vi "test_libssh2_sftp_readlink.vi"() -> ()   [LabVIEW 2017, in "integration_tests.lvlib"]
uses:
  integration_tests.lvlib
  libssh2/libssh2_sftp_symlink_ex.vi
  support/support.lvlib
  libssh2/libssh2.lvlib
  <vilib>/PNR/Transparent Assertions/Transparent Assertions/Transparent Assertions.lvlib
panel:
  out "error out":errorcluster
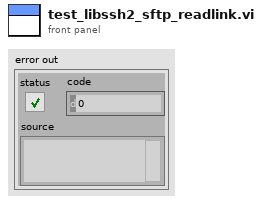
[diagram p1: front panel]
types:
  T1 = typedef "libssh2.lvlib/Session Refnum.ctl" = refnum<k1>
  T2 = typedef "libssh2.lvlib/SFTP Refnum.ctl" = refnum<k1>
  T3 = typedef "libssh2.lvlib/SFTP Handle Refnum.ctl" = refnum<k1>
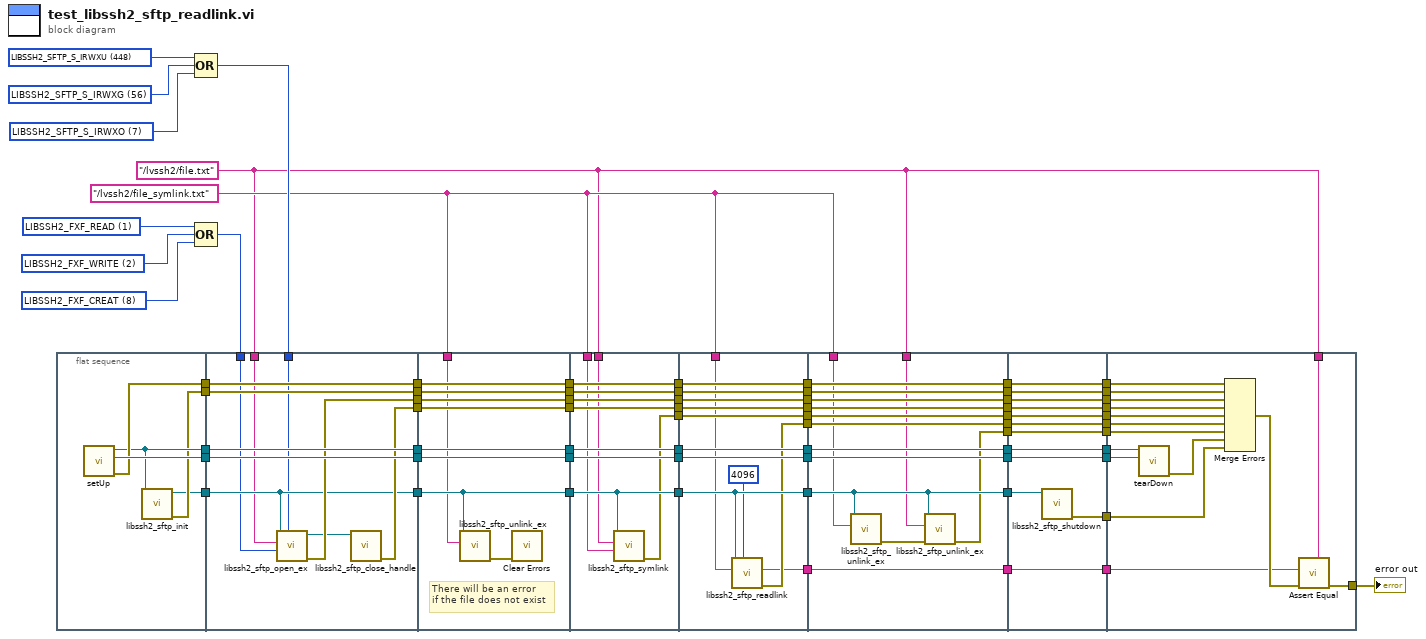
[diagram p0: block diagram]
diagram:
  w4 = "/lvssh2/file_symlink.txt" ("filename")
  w59 = u32 2 items=["LIBSSH2_FXF_READ"=1, "LIBSSH2_FXF_WRITE"=2, "LIBSSH2_FXF_APPEND"=4, "LIBSSH2_FXF_CREAT"=8, "LIBSSH2_FXF_TRUNC"=16, "LIBSSH2_FXF_EXCL"=32] ("flags")
  w60 = u32 1 items=["LIBSSH2_FXF_READ"=1, "LIBSSH2_FXF_WRITE"=2, "LIBSSH2_FXF_APPEND"=4, "LIBSSH2_FXF_CREAT"=8, "LIBSSH2_FXF_TRUNC"=16, "LIBSSH2_FXF_EXCL"=32] ("flags")
  w58 = u32 8 items=["LIBSSH2_FXF_READ"=1, "LIBSSH2_FXF_WRITE"=2, "LIBSSH2_FXF_APPEND"=4, "LIBSSH2_FXF_CREAT"=8, "LIBSSH2_FXF_TRUNC"=16, "LIBSSH2_FXF_EXCL"=32] ("flags")
  w3 = "/lvssh2/file.txt" ("filename")
  w62 = 7 items=["LIBSSH2_SFTP_S_IRWXU"=448, "LIBSSH2_SFTP_S_IRUSR"=256, "LIBSSH2_SFTP_S_IWUSR"=128, "LIBSSH2_SFTP_S_IXUSR"=64, "LIBSSH2_SFTP_S_IRWXG"=56, "LIBSSH2_SFTP_S_IRGRP"=32, "LIBSSH2_SFTP_S_IWGRP"=16, "LIBSSH2_SFTP_S_IXGRP"=8, "LIBSSH2_SFTP_S_IRWXO"=7, "LIBSSH2_SFTP_S_IROTH"=4, "LIBSSH2_SFTP_S_IWOTH"=2, "LIBSSH2_SFTP_S_IXOTH"=1] ("mode")
  w63 = 56 items=["LIBSSH2_SFTP_S_IRWXU"=448, "LIBSSH2_SFTP_S_IRUSR"=256, "LIBSSH2_SFTP_S_IWUSR"=128, "LIBSSH2_SFTP_S_IXUSR"=64, "LIBSSH2_SFTP_S_IRWXG"=56, "LIBSSH2_SFTP_S_IRGRP"=32, "LIBSSH2_SFTP_S_IWGRP"=16, "LIBSSH2_SFTP_S_IXGRP"=8, "LIBSSH2_SFTP_S_IRWXO"=7, "LIBSSH2_SFTP_S_IROTH"=4, "LIBSSH2_SFTP_S_IWOTH"=2, "LIBSSH2_SFTP_S_IXOTH"=1] ("mode")
  w64 = 448 items=["LIBSSH2_SFTP_S_IRWXU"=448, "LIBSSH2_SFTP_S_IRUSR"=256, "LIBSSH2_SFTP_S_IWUSR"=128, "LIBSSH2_SFTP_S_IXUSR"=64, "LIBSSH2_SFTP_S_IRWXG"=56, "LIBSSH2_SFTP_S_IRGRP"=32, "LIBSSH2_SFTP_S_IWGRP"=16, "LIBSSH2_SFTP_S_IXGRP"=8, "LIBSSH2_SFTP_S_IRWXO"=7, "LIBSSH2_SFTP_S_IROTH"=4, "LIBSSH2_SFTP_S_IWOTH"=2, "LIBSSH2_SFTP_S_IXOTH"=1] ("mode")
  n1 = flat-sequence {
    tunnel: [w73] -> w70
    tunnel: [w75] -> w69
    tunnel: [w74] -> w68
    tunnel: [w72] -> w66
    tunnel: [w71] -> w65
    tunnel: [w86] -> w38
    tunnel: [w85] -> w36
    tunnel: [w80] -> w34
    tunnel: [w84] -> w32
    tunnel: [w83] -> w30
    tunnel: [w82] -> w28
    tunnel: [w81] -> w26
    tunnel: w57 -> [w77]
    tunnel: w3 -> [w78]
    tunnel: w61 -> [w79]
    tunnel: w65 -> [w80]
    tunnel: w66 -> [w83]
    tunnel: w68 -> [w84]
    tunnel: w69 -> [w85]
    tunnel: w70 -> [w86]
    tunnel: w38 -> [w95]
    tunnel: [w95] -> w37
    tunnel: w36 -> [w94]
    tunnel: [w94] -> w35
    tunnel: w34 -> [w88]
    tunnel: [w88] -> w33
    tunnel: w32 -> [w93]
    tunnel: [w93] -> w31
    tunnel: w30 -> [w92]
    tunnel: [w92] -> w29
    tunnel: w28 -> [w91]
    tunnel: [w91] -> w27
    tunnel: w26 -> [w90]
    tunnel: [w90] -> w25
    tunnel: w4 -> [w87]
    tunnel: w37 -> [w105]
    tunnel: [w105] -> w48
    tunnel: w35 -> [w104]
    tunnel: [w104] -> w47
    tunnel: w33 -> [w101]
    tunnel: [w101] -> w46
    tunnel: w31 -> [w103]
    tunnel: [w103] -> w45
    tunnel: w29 -> [w102]
    tunnel: [w102] -> w44
    tunnel: w3 -> [w97]
    tunnel: w4 -> [w98]
    tunnel: w27 -> [w100]
    tunnel: [w100] -> w43
    tunnel: w25 -> [w99]
    tunnel: [w99] -> w42
    tunnel: [w96] -> w41
    tunnel: w48 -> [w117]
    tunnel: [w117] -> w24
    tunnel: w47 -> [w116]
    tunnel: [w116] -> w22
    tunnel: w46 -> [w110]
    tunnel: [w110] -> w20
    tunnel: [w107] -> w18
    tunnel: w45 -> [w115]
    tunnel: [w115] -> w16
    tunnel: w44 -> [w114]
    tunnel: [w114] -> w14
    tunnel: w43 -> [w113]
    tunnel: [w113] -> w12
    tunnel: w42 -> [w112]
    tunnel: [w112] -> w10
    tunnel: w41 -> [w111]
    tunnel: [w111] -> w8
    tunnel: w4 -> [w109]
    tunnel: [w108] -> w6
    tunnel: w24 -> [w131]
    tunnel: [w131] -> w23
    tunnel: w22 -> [w130]
    tunnel: [w130] -> w21
    tunnel: w20 -> [w122]
    tunnel: [w122] -> w19
    tunnel: w18 -> [w129]
    tunnel: [w129] -> w17
    tunnel: w16 -> [w128]
    tunnel: [w128] -> w15
    tunnel: w14 -> [w127]
    tunnel: [w127] -> w13
    tunnel: w12 -> [w126]
    tunnel: [w126] -> w11
    tunnel: w10 -> [w125]
    tunnel: [w125] -> w9
    tunnel: w8 -> [w124]
    tunnel: [w124] -> w7
    tunnel: w6 -> [w123]
    tunnel: [w123] -> w5
    tunnel: w4 -> [w121]
    tunnel: w3 -> [w120]
    tunnel: [w118] -> w2
    tunnel: w23 -> [w143]
    tunnel: [w143] -> w56
    tunnel: w21 -> [w142]
    tunnel: [w142] -> w55
    tunnel: w19 -> [w138]
    tunnel: w17 -> [w141]
    tunnel: [w141] -> w54
    tunnel: w15 -> [w140]
    tunnel: [w140] -> w53
    tunnel: w13 -> [w139]
    tunnel: [w139] -> w52
    tunnel: [w137] -> w51
    tunnel: w11 -> [w136]
    tunnel: [w136] -> w50
    tunnel: w9 -> [w135]
    tunnel: [w135] -> w49
    tunnel: w7 -> [w134]
    tunnel: [w134] -> w40
    tunnel: w5 -> [w133]
    tunnel: [w133] -> w39
    tunnel: w2 -> [w132]
    tunnel: [w132] -> w1
    tunnel: w56 -> [w158]
    tunnel: w55 -> [w157]
    tunnel: w54 -> [w146]
    tunnel: w53 -> [w156]
    tunnel: [w153] -> w67
    tunnel: w52 -> [w152]
    tunnel: w51 -> [w151]
    tunnel: w50 -> [w150]
    tunnel: w49 -> [w149]
    tunnel: w40 -> [w148]
    tunnel: w39 -> [w147]
    tunnel: w3 -> [w145]
    tunnel: w1 -> [w144]
    frame #0 {
      n2 = call "setUp.vi"() -> ("error out"=w74:errorcluster, "connection ID"=w75:refnum<k5>, "session"=w73:T1)  [unwired: 9 in]
      n3 = call "libssh2_sftp_init.vi"("session"=w73) -> ("error out"=w72:errorcluster, "sftp"=w71:T2)  [unwired: 9 in]
    }
    frame #1 {
      n4 = call "libssh2_sftp_open_ex.vi"("mode"=w79, "flags"=w77, "filename"=w78, "sftp"=w80) -> ("error out"=w82:errorcluster, "sftp handle"=w76:T3)  [unwired: 6 in]
      n5 = call "libssh2_sftp_close_handle.vi"("sftp handle"=w76) -> ("error out"=w81:errorcluster)  [unwired: 10 in]
    }
    frame #2 {
      # "There will be an error\nif the file does not exist"
      n6 = call "libssh2_sftp_unlink_ex.vi"("file"=w87, "sftp"=w88) -> ("error out"=w89:errorcluster)  [unwired: 9 in]
      n7 = call <vilib>:"Clear Errors.vi"("error in (no error)"=w89) -> ()  [unwired: 5 in, 2 out]
    }
    frame #3 {
      n8 = call "libssh2_sftp_symlink.vi"("target"=w98, "path"=w97, "sftp"=w101) -> ("error out"=w96:errorcluster)  [unwired: 8 in]
    }
    frame #4 {
      n9 = call "libssh2_sftp_readlink.vi"("maxlen"=u32 4096, "path"=w109, "sftp"=w110) -> ("error out"=w108:errorcluster, "target"=w107:string)  [unwired: 7 in]
    }
    frame #5 {
      n10 = call "libssh2_sftp_unlink_ex.vi"("file"=w121, "sftp"=w122) -> ("error out"=w119:errorcluster)  [unwired: 9 in]
      n11 = call "libssh2_sftp_unlink_ex.vi"("error in (no error)"=w119, "file"=w120, "sftp"=w122) -> ("error out"=w118:errorcluster)  [unwired: 8 in]
    }
    frame #6 {
      n12 = call "libssh2_sftp_shutdown.vi"("sftp"=w138) -> ("error out"=w137:errorcluster)  [unwired: 10 in]
    }
    frame #7 {
      n13 = call "tearDown.vi"("connection ID"=w157, "session"=w158) -> ("error out"=w155:errorcluster)  [unwired: 9 in]
      n14 = Merge Errors(w156, w152, w150, w149, w148, w147, w144, w155, w151) -> (w154:errorcluster)
      n15 = call <vilib>:"Assert Equal.vi"("Expected"=w145, "error in (no error)"=w154, "Actual"=w146) -> ("error out"=w153:errorcluster)  [unwired: 8 in]
    }
  }
  n16 = Compound Arithmetic op=OR(w64, w63, w62) -> (w61:i32)
  n17 = Compound Arithmetic op=OR(w60, w59, w58) -> (w57:u32)
  "error out" <- w67
